vi "Display Module - Remove Bad Refs.vi"(7 "Image Refs In":T1[](array[typedef])) -> (8 "Image Refs Out":T1[](array[typedef]))   [LabVIEW 2021]
uses:
  <vilib>/vision/Image Controls.llb/IMAQ Image.ctl
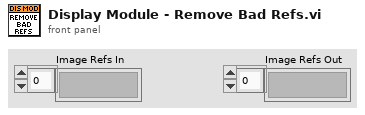
[diagram p1: front panel]
types:
  T1 = typedef "IMAQ Image.ctl" = refnum<image>
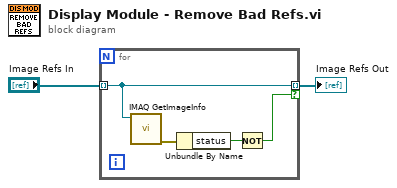
[diagram p0: block diagram]
diagram:
  n1 = for {
    tunnel: "Image Refs In" -> [w5] mode=indexing
    tunnel: [w5] -> w1 mode=indexing if=w3
    n2 = call "IMAQ GetImageInfo"("Image"=w5) -> ("error out"=w6:errorcluster)  [unwired: 3 in, 7 out]
    n3 = Unbundle By Name(w6) -> ("status"=w4:bool)
    n4 = Not(x=w4) -> (.not. x?=w3:bool)
  }
  "Image Refs Out" <- w1
